vi "Limit Control.vi"(9 "Numeric":dbl) -> (1 "Numeric 2":dbl)   [LabVIEW 2013]
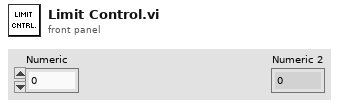
[diagram p1: front panel]
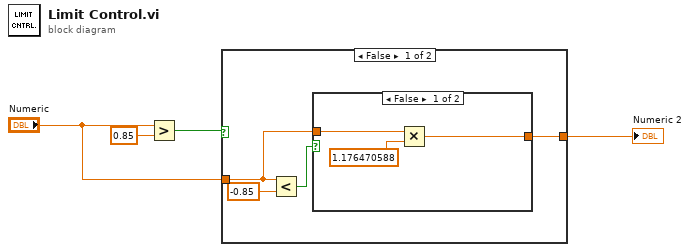
[diagram p0: block diagram]
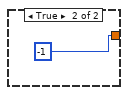
[diagram p2: hidden frame]
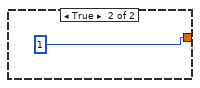
[diagram p3: hidden frame]
diagram:
  n1 = Greater?(x="Numeric", y=0.85) -> (0:w4:bool)
  n2 = case shown="False" w4 {
    tunnel: "Numeric" -> [w6 _]
    tunnel: [w5 1] -> w1
    frame False {
      n3 = Less?(x=w6, y=-0.85) -> (x < y?=w7:bool)
      n4 = case shown="False" w7 {
        tunnel: w6 -> [w10 _]
        tunnel: [w9 -1] -> w5
        frame False {
          n5 = Multiply(x=w10, y=1.176470588) -> (x*y=w9:dbl)
        }
        frame True {
        }
      }
    }
    frame True {
    }
  }
  "Numeric 2" <- w1
